vi "SelectChargeStateDC.vi"(8 "error in (no error)":errorcluster, 10 "Unique Object Identifier":string, 11 "DataCollector in":refnum<class "DataCollector.lvclass">) -> (0 "error out":errorcluster, 2 "Charge State":T1, 3 "DataCollector out":refnum<class "DataCollector.lvclass">)   [LabVIEW 2017, in "DataCollector.lvclass"]
uses:
  DataCollector.lvclass
  DataCollector.lvclass/DataCollector.ctl
  <vilib>/drjdpowell/SQLite Library/SQL Statement/SQL Statement.lvclass/SQL Statement.ctl
  <vilib>/drjdpowell/SQLite Library/SQL Statement/Column I64.vi
  <vilib>/drjdpowell/SQLite Library/SQL Statement/Column DBL.vi
  <vilib>/drjdpowell/SQLite Library/SQL Statement/Step.vi
  <vilib>/drjdpowell/SQLite Library/SQL Statement/Column Type.vi
  <vilib>/drjdpowell/SQLite Library/SQL Statement/Error Message.vi
  <vilib>/drjdpowell/SQLite Library/SQL Statement/SQL Statement.lvclass
  <vilib>/drjdpowell/SQLite Library/SQL Connection/Connection.lvclass
panel:
  out "concatenated string":string
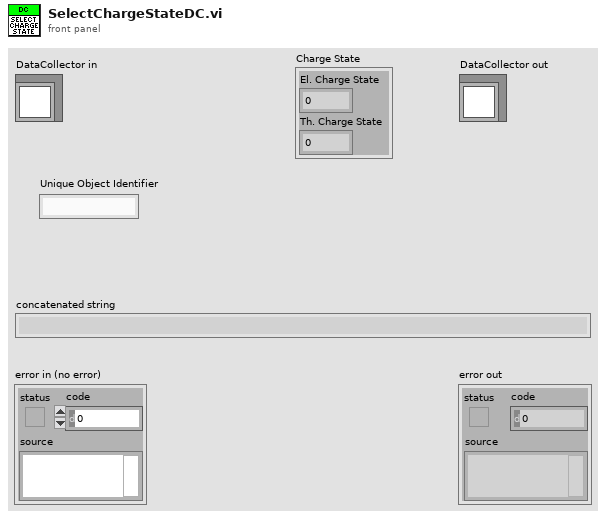
[diagram p1: front panel]
types:
  T1 = cluster{"El. Charge State":dbl, "Th. Charge State":dbl}
  T2 = cluster{"Column:Get Column DBL":dbl, "Column:Get Column DBL":dbl}
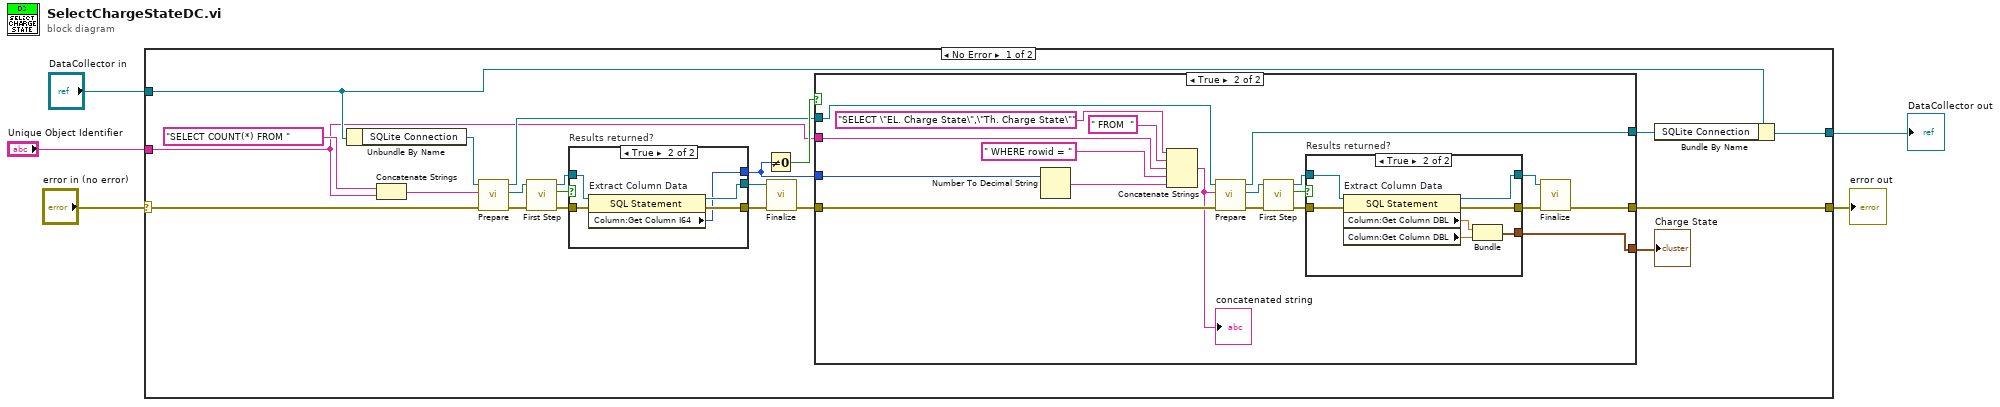
[diagram p0: block diagram]
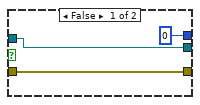
[diagram p2: hidden frame]
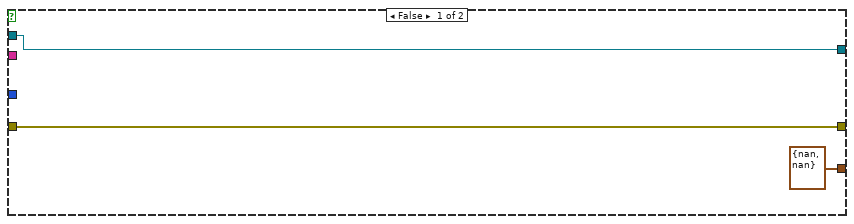
[diagram p3: hidden frame]
diagram:
  n1 = case shown="No Error" "error in (no error)" {
    selector: "error in (no error)" -> [w9 w67]
    tunnel: [w24 w67] -> w3
    tunnel: [w25 w66] -> w4
    tunnel: "DataCollector in" -> [w26 w66]
    tunnel: "Unique Object Identifier" -> [w7 _]
    frame No Error {
      n2 = Unbundle By Name(w26) -> ("SQLite Connection"=w13:refnum<class "Connection.lvclass">)
      n3 = Concatenate Strings("SELECT COUNT(*) FROM " ("String"), w7) -> (w6:string)
      n4 = call <vilib>:"Prepare.vi"("error in (no error)"=w9, "SQL"=w6, "SQLite Connection in"=w13) -> ("error out"=w14:errorcluster, "SQL Statement out"=w15:refnum<class "SQL Statement.lvclass">, "SQLite Connection out"=w12:refnum<class "Connection.lvclass">)  [unwired: 4 in, 2 out]
      n5 = call <vilib>:"First Step.vi"("error in (no error)"=w14, "SQL Statement in"=w15) -> ("error out"=w16:errorcluster, "Row returned"=w18:bool, "SQL Statement out"=w17:refnum<class "SQL Statement.lvclass">)  [unwired: 7 in]
      n6 = case "Results returned?" shown="True" w18 {
        tunnel: [w29 w31] -> w20
        tunnel: [w28 w32] -> w19
        tunnel: w17 -> [w29 w34]
        tunnel: w16 -> [w28 w33]
        tunnel: [i64 0 ("Column:Get Column I64") w30] -> w11
        frame False {
        }
        frame True {
          n7 = property on="Extract Column Data" class="SQL Statement"(reference=w34, error in=w33) -> (reference out=w31:refnum<class "SQL Statement.lvclass">, error out=w32:errorcluster, "Column:Get Column I64"=w30:i64)
        }
      }
      n8 = Not Equal To 0?(x=w11) -> (x != 0?=w21:bool)
      n9 = call <vilib>:"Finalize.vi"("error in (no error)"=w19, "SQL Statement in"=w20) -> ("error out"=w10:errorcluster)  [unwired: 9 in]
      n10 = case shown="True" w21 {
        tunnel: [w36 w56] -> w24
        tunnel: w12 -> [w35 w53]
        tunnel: [w35 w52] -> w23
        tunnel: w10 -> [w36 w47]
        tunnel: [T2 {"Column:Get Column DBL"=nan, "Column:Get Column DBL"=nan} w45] -> w22
        tunnel: w11 -> [_ w44]
        tunnel: w7 -> [_ w41]
        frame False {
        }
        frame True {
          n11 = Number To Decimal String(number=w44) -> (decimal integer string=w38:string)  [unwired: 1 in]
          n12 = Concatenate Strings("SELECT \"EL. Charge State\",\"Th. Charge State\"" ("string"), " FROM  " ("string"), w41, " WHERE rowid = " ("string"), w38) -> (w40:string)
          "concatenated string" <- w40
          n13 = call <vilib>:"Prepare.vi"("error in (no error)"=w47, "SQL"=w40, "SQLite Connection in"=w53) -> ("error out"=w55:errorcluster, "SQL Statement out"=w54:refnum<class "SQL Statement.lvclass">, "SQLite Connection out"=w52:refnum<class "Connection.lvclass">)  [unwired: 4 in, 2 out]
          n14 = call <vilib>:"First Step.vi"("error in (no error)"=w55, "SQL Statement in"=w54) -> ("error out"=w51:errorcluster, "Row returned"=w49:bool, "SQL Statement out"=w50:refnum<class "SQL Statement.lvclass">)  [unwired: 7 in]
          n15 = case "Results returned?" shown="True" w49 {
            tunnel: [w58 w62] -> w46
            tunnel: [w57 w63] -> w48
            tunnel: w50 -> [w58 w65]
            tunnel: w51 -> [w57 w64]
            tunnel: [_ w59] -> w45
            frame False {
            }
            frame True {
              n16 = property on="Extract Column Data" class="SQL Statement"(reference=w65, error in=w64) -> (reference out=w62:refnum<class "SQL Statement.lvclass">, error out=w63:errorcluster, "Column:Get Column DBL"=w61:dbl, "Column:Get Column DBL"=w60:dbl)
              n17 = Bundle("Column:Get Column DBL"=w61, "Column:Get Column DBL"=w60) -> (w59:T2)  [unwired: 1 in]
            }
          }
          n18 = call <vilib>:"Finalize.vi"("error in (no error)"=w48, "SQL Statement in"=w46) -> ("error out"=w56:errorcluster)  [unwired: 9 in]
        }
      }
      "Charge State" <- w22
      n19 = Bundle By Name(cluster=w26, "SQLite Connection"=w23) -> (w25:refnum<class "DataCollector.lvclass">)
    }
    frame Error {
    }
  }
  "error out" <- w3
  "DataCollector out" <- w4
